vi "Auto Griddy Score v2.vi"(8 "Command Info In":T2, 10 "intake modes":T1, 11 "Griddy Command":T5) -> (0 "Command Info Out":T2)   [LabVIEW 2020]
uses:
  Implementation/Typedefs/Teleop Manipulator Commands.ctl
  <vilib>/Rock Robotics/WPI/Framework/Command Status Info.ctl
  <vilib>/Rock Robotics/WPI/Framework/Completion Status.ctl
  <vilib>/Rock Robotics/WPI/Framework/Completion Notifier.ctl
  intake sub/Implementation/Typedef/intake typedef.ctl
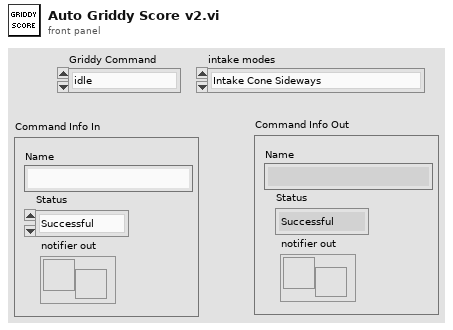
[diagram p1: front panel]
types:
  T1 = typedef "intake typedef.ctl" = enum16{"Intake Cone Sideways", "Intake Cone Upright", "Intake Cube", "Outtake/Score", "Shoot"}
  T2 = typedef "Command Status Info.ctl" = cluster{"Name":string, "Status":T3, "notifier out":T4}
  T3 = typedef "Completion Status.ctl" = enum16{"Successful", "Aborted", "Incomplete"}
  T4 = typedef "Completion Notifier.ctl" = refnum<notifier>
  T5 = typedef "Teleop Manipulator Commands.ctl" = enum16{"idle", "intake cone sideways", "intake cone upright", "intake cone feeder", "intake cube feeder", "intake cube", "score low cone", "score low cube", "score mid cone", "score mid cube", "score high cone", "score high cube", "score mid cone up"}
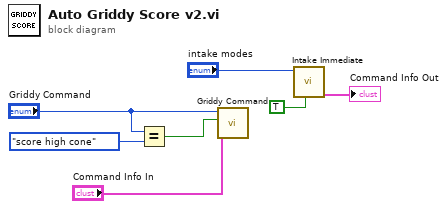
[diagram p0: block diagram]
diagram:
  n1 = Equal?(x="Griddy Command", y=Teleop_Manipulator_Commands."score high cone") -> (x = y?=w3:bool)
  n2 = call "Griddy Command.vi"("Command Info In"="Command Info In", "Flip Wrist"=w3, "Griddy Command"="Griddy Command") -> ()  [unwired: 8 in, 1 out]
  n3 = call "Intake Immediate.vi"("Wait for Manipulator"=TRUE, "intake modes"="intake modes") -> ("Command Info Out"=→"Command Info Out":T2)  [unwired: 9 in]
